vi "Read Board Game Vals.vi"(8 "error in (no error)":errorcluster, 11 "Board Game in":refnum<class "Board Game.lvclass">) -> (0 "error out":errorcluster, 2 "Board Game Vals":refnum<data-value>, 3 "Board Game out":refnum<class "Board Game.lvclass">)   [LabVIEW 2021, in "Board Game.lvclass"]
uses:
  Board Game.lvclass
  Board Game.lvclass/Board Game.ctl
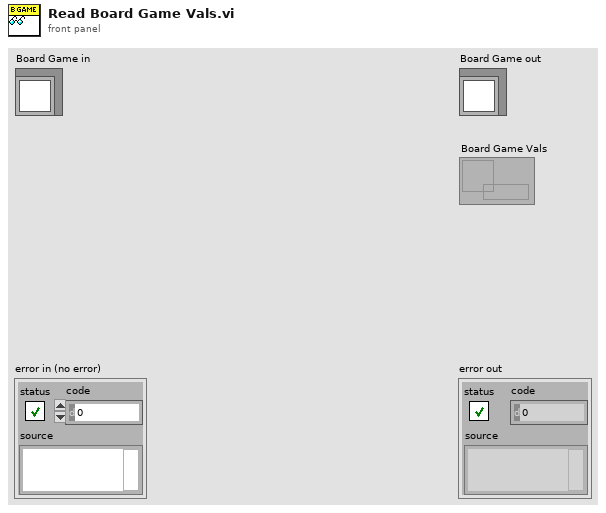
[diagram p1: front panel]
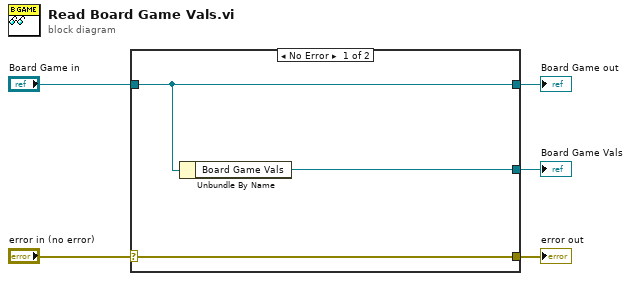
[diagram p0: block diagram]
diagram:
  n1 = case shown="No Error" "error in (no error)" {
    selector: "error in (no error)" -> [w8 w9]
    tunnel: [w8 w9] -> w4
    tunnel: [w7 w10] -> w2
    tunnel: "Board Game in" -> [w7 w10]
    tunnel: [w6 _] -> w1
    frame No Error {
      n2 = Unbundle By Name(w7) -> ("Board Game Vals"=w6:refnum<data-value>)
    }
    frame Error {
    }
  }
  "error out" <- w4
  "Board Game out" <- w2
  "Board Game Vals" <- w1
